vi "ConfigureHwChannels.vi"(8 "error in (no error)":errorcluster, 11 "config":T1) -> (0 "error out":errorcluster, 1 "valid":bool, 2 "register sweeps":T4[](array[typedef]), 3 "config out":T1)   [LabVIEW 2017, in "EmsaAcquisition.lvlib"]
uses:
  <vilib>/addons/InsightCM/Devices/Shared/Emsa/EmsaAcquisition/EmsaAcquisition.lvlib
  <vilib>/addons/InsightCM/Devices/Shared/Emsa/EmsaDataEventCreator/controls/RegisterSweepRoutedMessage.ctl
  <vilib>/addons/InsightCM/Devices/Shared/Emsa/EmsaDataEventCreator/controls/Registry_Sweep.ctl
  <vilib>/addons/InsightCM/Devices/Shared/Common/DataEvent/controls/DataSetType.ctl
  <vilib>/addons/InsightCM/MessageBus/Base/controls/KeyValuePair.ctl
  <vilib>/addons/InsightCM/Devices/Shared/Emsa/EmsaAcquisition/controls/config.ctl
  <vilib>/addons/InsightCM/Devices/Shared/Emsa/Emsa9770API/9770 API.lvclass
  <vilib>/addons/InsightCM/Devices/Shared/Emsa/EmsaAcquisition/controls/group.ctl
  <vilib>/addons/InsightCM/Devices/Shared/Emsa/EmsaAcquisition/controls/acqConfig.ctl
  <vilib>/addons/InsightCM/Utilities/DeviceModelHelpers/DeviceModelHelpers.lvlib
  <vilib>/addons/InsightCM/Utilities/GlobalConfiguration/GlobalConfiguration.lvlib
  <vilib>/addons/InsightCM/Utilities/PropertyHelpers/PropertyHelpers.lvlib
  <vilib>/addons/InsightCM/Devices/Shared/Common/DataEvent/DataEvent.lvlib
  <vilib>/addons/InsightCM/Devices/Shared/Emsa/EmsaDataEventCreator/EmsaDataEventCreator.lvlib
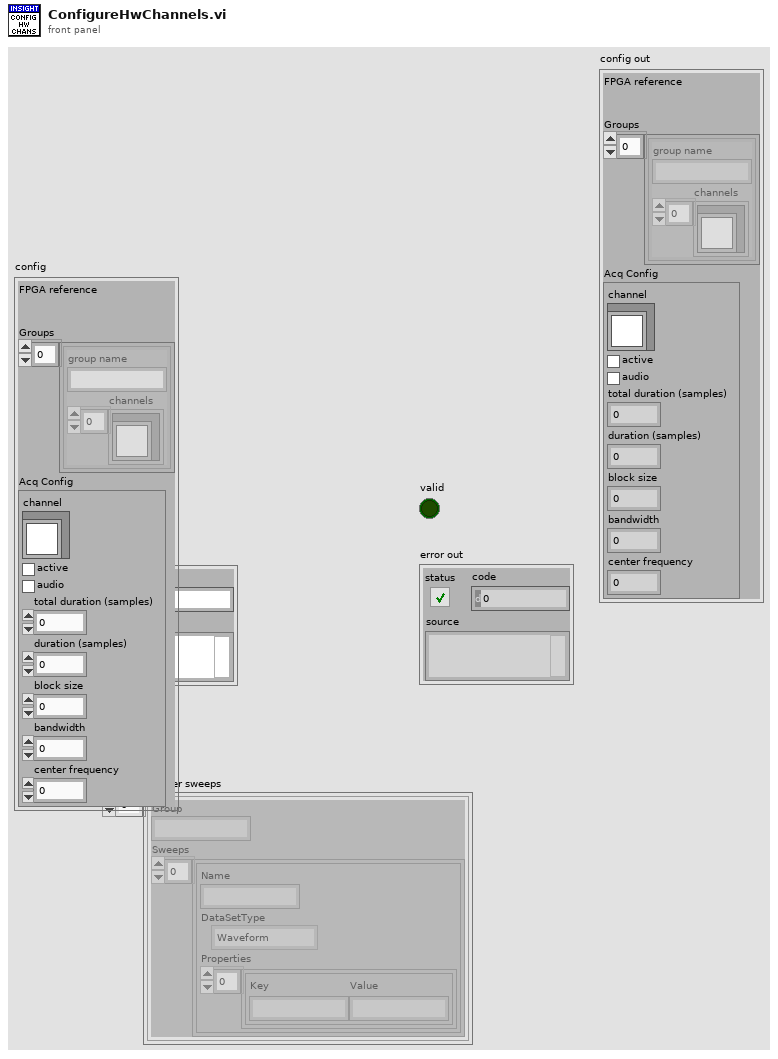
[diagram p1: front panel]
types:
  T1 = typedef "EmsaAcquisition.lvlib/config.ctl" = cluster{"FPGA reference":refnum<k20>, "Groups":T2[], "Acq Config":T3}
  T2 = typedef "EmsaAcquisition.lvlib/group.ctl" = cluster{"group name":string, "channels":refnum<class "9770 API.lvclass">[]}
  T3 = typedef "EmsaAcquisition.lvlib/acqConfig.ctl" = cluster{"channel":refnum<class "9770 API.lvclass">, "active":bool, "audio":bool, "total duration (samples)":i32, "duration (samples)":i32, "block size":i32, "bandwidth":dbl, "center frequency":dbl}
  T4 = typedef "EmsaDataEventCreator.lvlib/RegisterSweepRoutedMessage.ctl" = cluster{"Group":string, "Sweeps":T5[]}
  T5 = typedef "EmsaDataEventCreator.lvlib/Registry_Sweep.ctl" = cluster{"Name":string, "DataSetType":T6, "Properties":T7[]}
  T6 = typedef "DataEvent.lvlib/DataSetType.ctl" = enum16{"Waveform", "SpeedProfile", "ThermalImage", "EmsaSweep"}
  T7 = typedef "KeyValuePair.ctl" = cluster{"Key":string, "Value":string}
  T8 = typedef "R2_DeviceModel.ctl" = cluster{"Device":T9, "Channels":T16[], "Tags":T18[]}
  T9 = typedef "R2_Device.ctl" = cluster{"Id":string, "Name":string, "DeviceType":string, "HardwareName":string, "IpAddress":string, "HardwareInfo":T7[], "ApplicationType":string, "ApplicationVersion":string, "EquipmentIds":string[], "ConfigurationVersion":string, "State":T10, "Properties":T7[], "DataGroups":T11[], "BurstModeTrigger":T15}
  T10 = typedef "DeviceState.ctl" = cluster{"Disabled":bool}
  T11 = typedef "R2_DataGroup.ctl" = cluster{"Name":string, "OperatingStates":T12[], "Properties":T7[], "EquipmentIds":string[], "AssetNodeId":string}
  T12 = typedef "OperatingState.ctl" = cluster{"Name":string, "Properties":T7[], "Triggers":T13[]}
  T13 = typedef "Trigger.ctl" = cluster{"Type":string, "Expression":string, "Conditions":T14[]}
  T14 = typedef "Condition.ctl" = cluster{"Source":string, "Type":string, "Operator":string, "CompareTo":string, "DwellSeconds":dbl}
  T15 = typedef "BurstModeTrigger.ctl" = cluster{"Trigger":T13, "SampleRate":string, "AcquisitionLength":string}
  T16 = typedef "R2_Channel.ctl" = cluster{"Id":string, "DeviceId":string, "Name":string, "ChannelType":string, "HardwareKey":string, "HardwareChannel":string, "DataGroup":string, "Keywords":string[], "EquipmentIds":string[], "Properties":T7[], "Metrics":T17[], "AssetNodeId":string, "MeasType":string, "AssetName":string}
  T17 = typedef "Metric.ctl" = cluster{"Id":string, "Name":string, "Unit":string, "Properties":T7[], "MetricDefinitionInstanceId":string}
  T18 = typedef "Tag.ctl" = cluster{"Id":string, "Path":string, "Name":string, "Datatype":string, "Props":T7[], "Keywords":string[]}
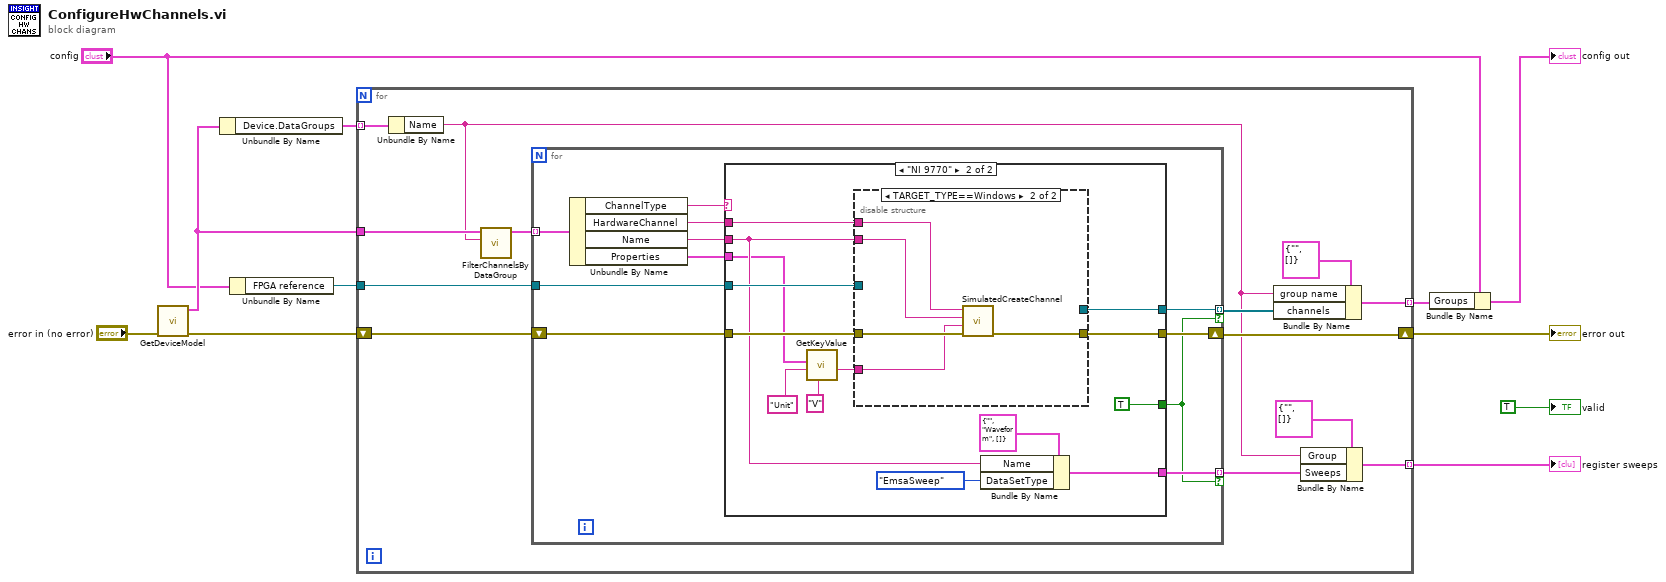
[diagram p0: block diagram]
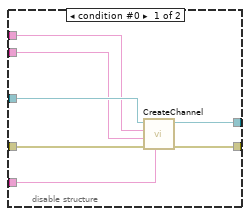
[diagram p3: hidden frame]
diagram:
  n1 = call <vilib>:"GetDeviceModel.vi"("error in (no error)"="error in (no error)") -> ("error out"=w6:errorcluster, "device model"=w7:T8)  [unwired: 8 in, 1 out]
  n2 = Unbundle By Name(w7) -> ("Device.DataGroups"=w10:T11[])
  n3 = Unbundle By Name("config") -> ("FPGA reference"=w4:refnum<k20>)
  n4 = for {
    tunnel: w10 -> [w24] mode=indexing
    tunnel: w7 -> [w23]
    tunnel: w4 -> [w22]
    shift-right: [w21] -> w8
    shift-left: w6 -> [w20]
    tunnel: [w17] -> w1 mode=indexing
    tunnel: [w15] -> w5 mode=indexing
    n5 = Unbundle By Name(w24) -> ("Name"=w16:string)
    n6 = call <vilib>:"FilterChannelsByDataGroup.vi"("group"=w16, "device model"=w23) -> ("channels in data group"=w19:T16[])  [unwired: 8 in, 1 out]
    n7 = for {
      tunnel: w19 -> [w35] mode=indexing
      tunnel: w22 -> [w34]
      shift-right: [w33] -> w21
      shift-left: w20 -> [w32]
      tunnel: [w28] -> w18 mode=indexing if=w26
      tunnel: [w27] -> w14 mode=indexing if=w26
      n8 = Unbundle By Name(w35) -> ("ChannelType"=w25:string, "HardwareChannel"=w31:string, "Name"=w30:string, "Properties"=w29:T7[])
      n9 = case shown="\"NI 9770\"" w25 {
        tunnel: w34 -> [_ w49]
        tunnel: w32 -> [w36 w50]
        tunnel: [w36 w43] -> w33
        tunnel: w31 -> [_ w48]
        tunnel: w30 -> [_ w46]
        tunnel: w29 -> [_ w42]
        tunnel: [_ w44] -> w28
        tunnel: [_ TRUE] -> w26
        tunnel: [_ w45] -> w27
        frame "", Default {
        }
        frame "NI 9770" {
          n10 = call <vilib>:"GetKeyValue.vi"("default value"="V", "key"="Unit", "key value pairs"=w42) -> ("value"=w41:string)  [unwired: 6 in, 2 out]
          n11 = disable-structure shown="TARGET_TYPE==Windows" {
            disable-tunnel: w50 -> [w57 w61]
            disable-tunnel: w49 -> [w56 _]
            disable-tunnel: w48 -> [w55 w58]
            disable-tunnel: w46 -> [w54 w59]
            disable-tunnel: [w53 _] -> w44
            disable-tunnel: [w52 w62] -> w43
            disable-tunnel: w41 -> [w51 w60]
            frame condition #0 {
              n12 = call <vilib>:"CreateChannel.vi"("Units"=w51, "error in (no error)"=w57, "ChannelName"=w54, "ChannelID"=w55, "FPGA reference"=w56) -> ("error out"=w52:errorcluster, "9770 API out"=w53:refnum<class "9770 API.lvclass">)  [unwired: 5 in]
            }
            frame condition #1 (active) {
              n13 = call <vilib>:"SimulatedCreateChannel.vi"("error in (no error)"=w61, "Unit"=w60, "Name"=w59, "HardwareChannel"=w58) -> ("error out"=w62:errorcluster)  [unwired: 7 in]
            }
          }
          n14 = Bundle By Name(cluster=T5 {"Name"="", "DataSetType"=enum."Waveform", "Properties"=[]} ("Sweep Registry"), "Name"=w46, "DataSetType"=DataSetType."EmsaSweep") -> (w45:T5)
        }
      }
    }
    n15 = Bundle By Name(cluster=T2 {"group name"="", "channels"=[]}, "group name"=w16, "channels"=w18) -> (w17:T2)
    n16 = Bundle By Name(cluster=T4 {"Group"="", "Sweeps"=[]} ("RegisterSweepRoutedMessage"), "Group"=w16, "Sweeps"=w14) -> (w15:T4)
  }
  "error out" <- w8
  "register sweeps" <- w5
  n17 = Bundle By Name(cluster="config", "Groups"=w1) -> (→"config out":T1)
  "valid" <- TRUE ("valid")
